vi "Close.vi"(8 "error in (no error)":errorcluster, 9 "Close after execution (F)?":bool, 11 "UI_Interaction_Manager in":refnum<class "UI_Interaction_Manager.lvclass">) -> (0 "error out":errorcluster)   [LabVIEW 2011, in "UI_Interaction_Manager.lvclass"]
uses:
  UI_Interaction_Manager.lvclass
  UI_Interaction_Manager.lvclass/UI_Interaction_Manager.ctl
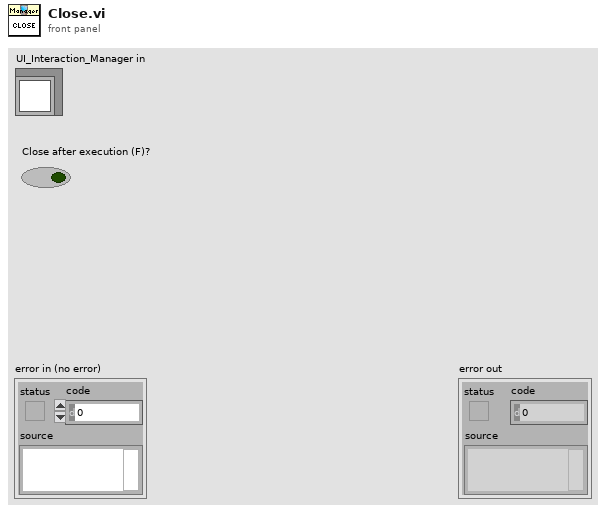
[diagram p1: front panel]
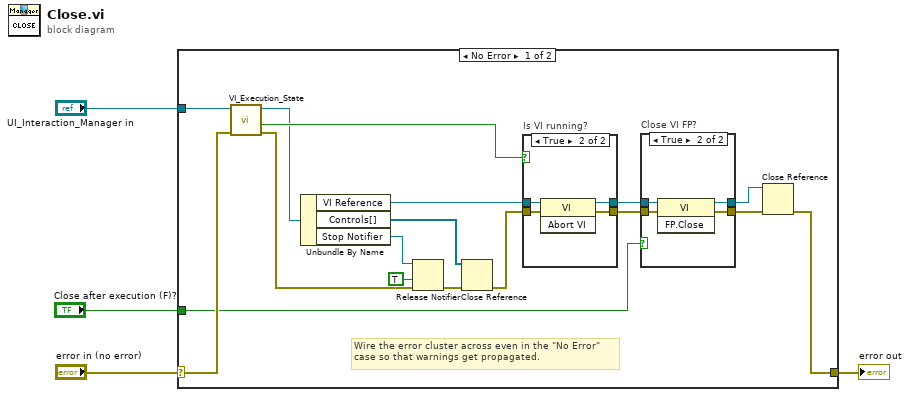
[diagram p0: block diagram]
diagram:
  n1 = case shown="No Error" "error in (no error)" {
    selector: "error in (no error)" -> [w19 w34]
    tunnel: [w21 w34] -> w3
    tunnel: "UI_Interaction_Manager in" -> [w20 _]
    tunnel: "Close after execution (F)?" -> [w14 _]
    frame No Error {
      # "Wire the error cluster across even in the \"No Error\"\ncase so that warnings get propagated."
      n2 = call "VI_Execution_State.vi"("error in (no error)"=w19, "UI_Interaction_Manager in"=w20) -> ("error out"=w10:errorcluster, "Running?"=w18:bool, "UI_Interaction_Manager out"=w13:refnum<class "UI_Interaction_Manager.lvclass">)  [unwired: 6 in, 1 out]
      n3 = Unbundle By Name(w13) -> ("VI Reference"=w17:refnum<vi>, "Controls[]"=w7:refnum<vi>[], "Stop Notifier"=w9:refnum<notifier>)
      n4 = Release Notifier(notifier=w9, force destroy? (F)=TRUE, error in (no error)=w10) -> (error out=w6:errorcluster)  [unwired: 2 out]
      n5 = Close Reference(reference=w7, error in (no error)=w6) -> (error out=w5:errorcluster)
      n6 = case "Is VI running?" shown="True" w18 {
        tunnel: w17 -> [w28 w32]
        tunnel: w5 -> [w29 w33]
        tunnel: [w29 w31] -> w15
        tunnel: [w28 w30] -> w16
        frame False {
        }
        frame True {
          n7 = invoke class="VI" method="Abort VI"(reference=w32, error in=w33) -> (reference out=w30:refnum<vi>, error out=w31:errorcluster)  [unwired: 1 in, 1 out]
        }
      }
      n8 = case "Close VI FP?" shown="True" w14 {
        tunnel: [w23 w27] -> w12
        tunnel: w16 -> [w22 w26]
        tunnel: w15 -> [w23 w25]
        tunnel: [w22 w24] -> w11
        frame False {
        }
        frame True {
          n9 = invoke class="VI" method="FP.Close"(reference=w26, error in=w25) -> (reference out=w24:refnum<vi>, error out=w27:errorcluster)  [unwired: 1 in, 1 out]
        }
      }
      n10 = Close Reference(reference=w11, error in (no error)=w12) -> (error out=w21:errorcluster)
    }
    frame Error {
    }
  }
  "error out" <- w3
